vi "Read Back Tunnel Internal TermRefs.vi"(8 "error in (no error)":errorcluster, 10 "element":string, 11 "CSM-Helper in":refnum<class "CSM-Helper.lvclass">) -> (0 "error out":errorcluster, 2 "Back Tunnels":T1, 3 "CSM-Helper out":refnum<class "CSM-Helper.lvclass">)   [LabVIEW 2017, in "CSM-Helper.lvclass"]
doc: "### Read Back Tunnel Internal TermRefs.vi\n\n-- <b>Controls</b> --\n- <b>element</b>:\n- <b>CSM-Helper in</b>: CSMHelper input\n\n-- <b>Indicators</b> --\n- <b>Back Tunnels</b>:\n- <b>CSM-Helper out</b>: CSMHelper output"
uses:
  CSM-Helper.lvclass
  CSM-Helper.lvclass/CSM-Helper.ctl
  Read Back Tunnels Refs.vi
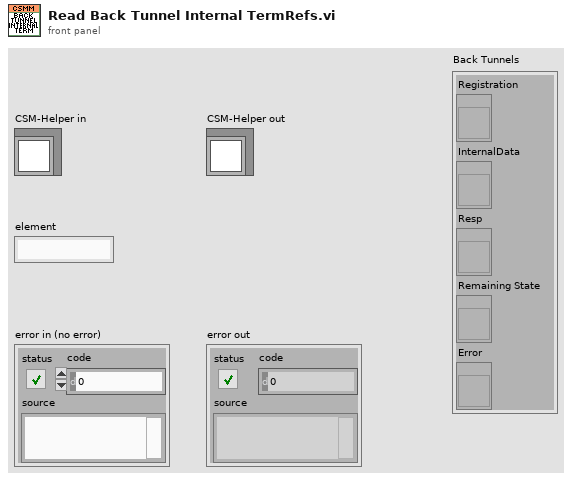
[diagram p1: front panel]
types:
  T1 = cluster{"Registration":refnum<vi>, "InternalData":refnum<vi>, "Resp":refnum<vi>, "Remaining State":refnum<vi>, "Error":refnum<vi>}
  T2 = typedef "CSM-Helper.lvclass/_csmhelper_Back_Tunnels_Refs.ctl" = cluster{"Registration":refnum<vi>, "InternalData":refnum<vi>, "Resp":refnum<vi>, "Remaining State":refnum<vi>, "Error":refnum<vi>}
  T3 = cluster{refnum<vi>, refnum<vi>, refnum<vi>, refnum<vi>, refnum<vi>}
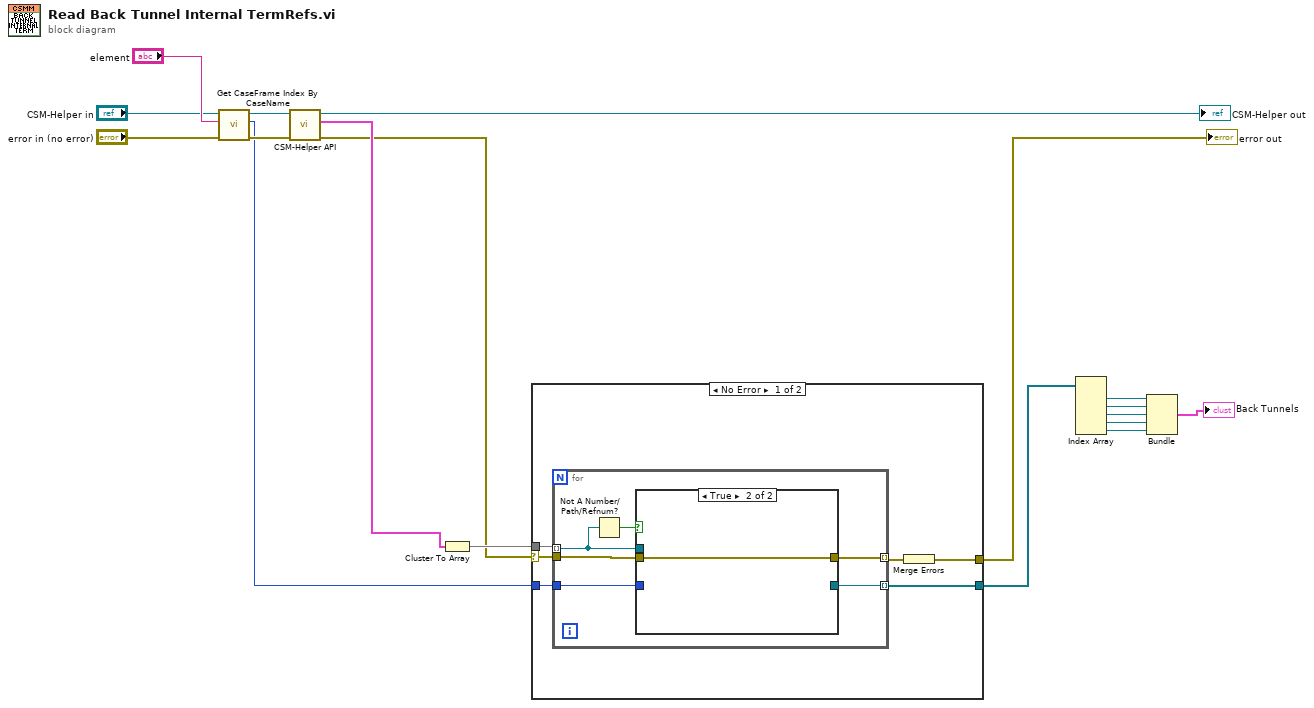
[diagram p0: block diagram]
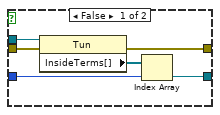
[diagram p2: hidden frame]
diagram:
  n1 = call "Get CaseFrame Index By CaseName.vi"("error in (no error)"="error in (no error)", "CASE"="element", "CSM-Helper in"="CSM-Helper in") -> ("error out"=w18:errorcluster, "index"=w5:i32, "CSM-Helper out"=w16:refnum<class "CSM-Helper.lvclass">)  [unwired: 5 in, 1 out]
  n2 = call-poly "CSM-Helper API.vi"("error in (no error)"=w18, "CSM-Helper in"=w16) -> ("error out"=w4:errorcluster, "Back Tunnels"=w6:T2, "CSM-Helper out"=→"CSM-Helper out":refnum<class "CSM-Helper.lvclass">)  [unwired: 7 in]
  n3 = Cluster To Array(cluster=w6) -> (array=w7:refnum<vi>[])
  n4 = case shown="No Error" w4 {
    selector: w4 -> [w20 w38]
    tunnel: [w24 _] -> w12
    tunnel: w7 -> [w22 _]
    tunnel: w5 -> [w21 _]
    tunnel: [w19 w38] -> w3
    frame No Error {
      n5 = for {
        tunnel: w21 -> [w30]
        tunnel: [w29] -> w24 mode=indexing
        tunnel: w22 -> [w26] mode=indexing
        tunnel: w20 -> [w28]
        tunnel: [w27] -> w23 mode=indexing
        n6 = Not A Number/Path/Refnum?(number/path/refnum=w26) -> (NaN/Path/Refnum?=w25:bool)
        n7 = case shown="True" w25 {
          tunnel: w30 -> [w35 _]
          tunnel: [w34 _] -> w29
          tunnel: w28 -> [w33 w37]
          tunnel: [w32 w37] -> w27
          tunnel: w26 -> [w31 _]
          frame False {
            n8 = property on="Property Node" class="Tun"(reference=w31, error in=w33) -> (error out=w32:errorcluster, "InsideTerms[]"=w36:refnum<vi>[])  [unwired: 1 out]
            n9 = Index Array(array=w36, index=w35) -> (element=w34:refnum<vi>)
          }
          frame True {
          }
        }
      }
      n10 = Merge Errors(w23) -> (w19:errorcluster)
    }
    frame Error {
    }
  }
  "error out" <- w3
  n11 = Index Array(array=w12) -> (element #1=w11:refnum<vi>, element #2=w10:refnum<vi>, element #3=w9:refnum<vi>, element #4=w8:refnum<vi>, element #5=w1:refnum<vi>)  [unwired: 5 in]
  n12 = Bundle(w11, w10, w9, w8, w1) -> (→"Back Tunnels":T3)  [unwired: 1 in]
